vi "AddOrReplaceCmdInCmdList.vi"(7 "CMD LUT in":variant, 8 "error in (no error)":errorcluster, 10 "New Command(s)":string, 11 "Command List In":string) -> (0 "error out":errorcluster, 3 "Command List Out":string, 5 "CMD LUT out":variant)   [LabVIEW 2026, in "MicroPulse_Driver.lvlib"]
uses:
  MicroPulse_Driver.lvlib
  <vilib>/Utility/error.llb/Trim Whitespace One-Sided.vi
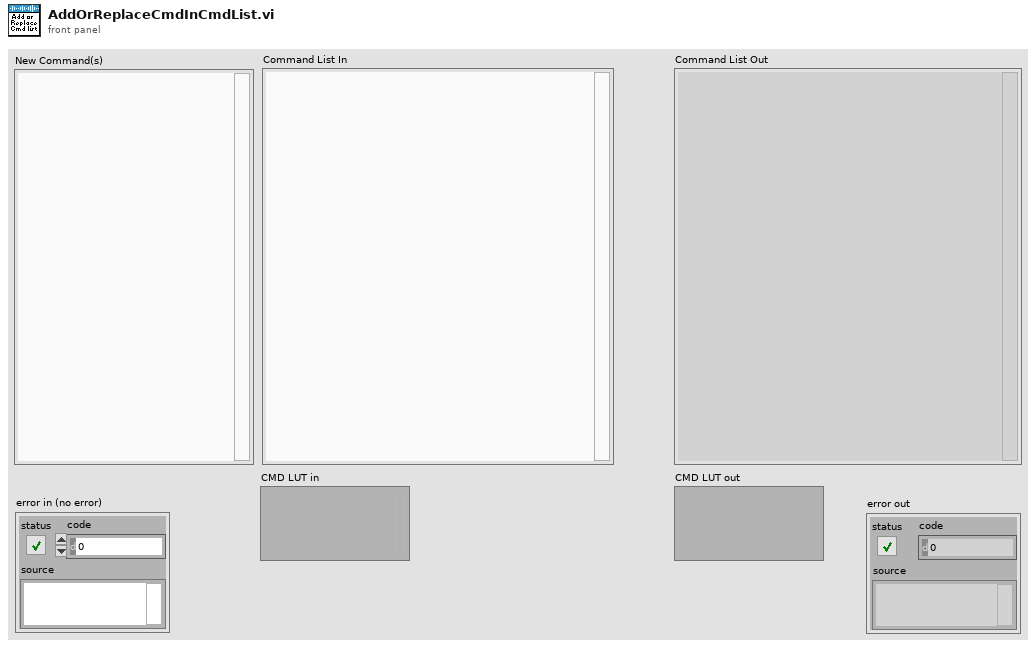
[diagram p1: front panel]
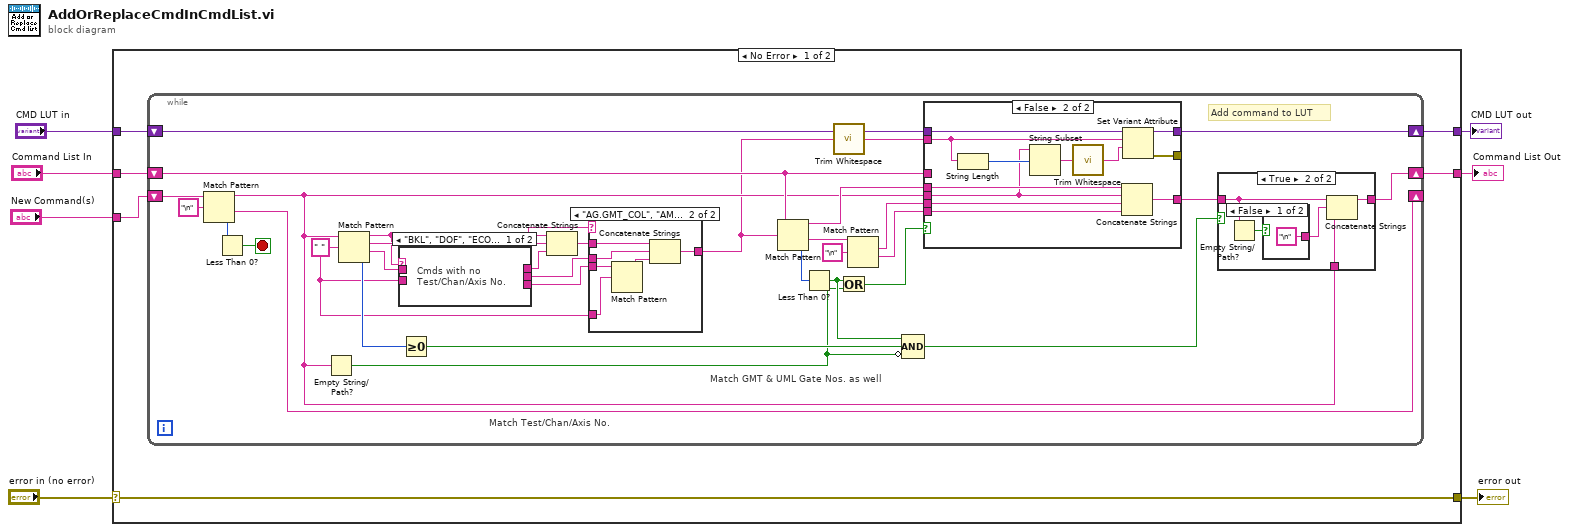
[diagram p0: block diagram]
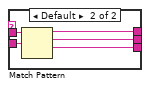
[diagram p2: hidden frame]
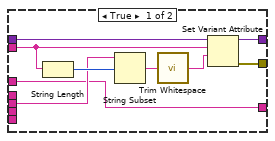
[diagram p6: hidden frame]
diagram:
  n1 = case shown="No Error" "error in (no error)" {
    selector: "error in (no error)" -> [w10 w89]
    tunnel: "Command List In" -> [w13 w88]
    tunnel: [w12 w88] -> w6
    tunnel: "New Command(s)" -> [w11 _]
    tunnel: [w10 w89] -> w3
    tunnel: "CMD LUT in" -> [w9 w87]
    tunnel: [w8 w87] -> w1
    frame No Error {
      n2 = while {
        shift-right: [w38] -> w12
        shift-left: w13 -> [w28]
        shift-right: [w27] -> _
        shift-left: w11 -> [w29]
        shift-right: [w17] -> w8
        shift-left: w9 -> [w18]
        stop <- w30 stop-if-true
        w20 = " " ("regular expression")
        # "Add command to LUT"
        # "Match GMT & UML Gate Nos. as well"
        # "Match Test/Chan/Axis No."
        n3 = Match Pattern(string=w29, regular expression="\n") -> (before substring=w22:string, after substring=w27:string, offset past match=w31:i32)  [unwired: 1 in, 1 out]
        n4 = Less Than 0?(x=w31) -> (x < 0?=w30:bool)
        n5 = Empty String/Path?(string/path=w22) -> (empty?=w34:bool)
        n6 = Match Pattern(string=w22, regular expression=w20) -> (before substring=w15:string, match substring=w24:string, after substring=w26:string, offset past match=w40:i32)  [unwired: 1 in]
        n7 = case shown="\"BKL\", \"DOF\", \"ECON\", \"EMUL\", \"ENCF\", \"ENCM\", \"ENCO\", \"ENCT\", \"FLM\", \"JIT\", \"MPE\", \"NUM\", \"PIG\", \"PRF\", \"SPA\", \"SPQ\", \"SPR\", \"STS\"" w15 {
          tunnel: w26 -> [_ w51]
          tunnel: [_ w50] -> w25
          tunnel: [_ w49] -> w21
          tunnel: w20 -> [_ w48]
          tunnel: [_ w47] -> w19
          frame "BKL", "DOF", "ECON", "EMUL", "ENCF", "ENCM", "ENCO", "ENCT", "FLM", "JIT", "MPE", "NUM", "PIG", "PRF", "SPA", "SPQ", "SPR", "STS" {
            # "Cmds with no\nTest/Chan/Axis No."
          }
          frame Default {
            n8 = Match Pattern(string=w51, regular expression=w48) -> (before substring=w50:string, match substring=w47:string, after substring=w49:string)  [unwired: 1 in, 1 out]
          }
        }
        n9 = Greater Or Equal To 0?(x=w40) -> (x >= 0?=w35:bool)
        n10 = Concatenate Strings(w15, w24, w25) -> (w23:string)
        n11 = case shown="\"AG.GMT_COL\", \"AMM\", \"CML\", \"GIN\", \"GMH\", \"GML\", \"GMT\", \"GTR\", \"HMS\", \"LML\", \"PMG\", \"UML\"" w15 {
          tunnel: [w52 w53] -> w16
          tunnel: w23 -> [w52 w56]
          tunnel: w21 -> [_ w58]
          tunnel: w20 -> [_ w57]
          tunnel: w19 -> [_ w55]
          frame Default {
          }
          frame "AG.GMT_COL", "AMM", "CML", "GIN", "GMH", "GML", "GMT", "GTR", "HMS", "LML", "PMG", "UML" {
            n12 = Match Pattern(string=w58, regular expression=w57) -> (before substring=w54:string)  [unwired: 1 in, 3 out]
            n13 = Concatenate Strings(w56, w55, w54) -> (w53:string)
          }
        }
        n14 = Match Pattern(string=w28, regular expression=w16) -> (before substring=w42:string, after substring=w46:string, offset past match=w41:i32)  [unwired: 1 in, 1 out]
        n15 = Less Than 0?(x=w41) -> (x < 0?=w36:bool)
        n16 = call <vilib>:"Trim Whitespace.vi"("string"=w16) -> ("trimmed string"=w14:string)  [unwired: 1 in]
        n17 = Or(x=w36, y=w34) -> (x .or. y?=w37:bool)
        n18 = Match Pattern(string=w46, regular expression="\n") -> (match substring=w44:string, after substring=w43:string)  [unwired: 1 in, 2 out]
        n19 = Compound Arithmetic op=AND(w36, w35, invert w34) -> (w33:bool)
        n20 = case shown="False" w37 {
          tunnel: w44 -> [_ w82]
          tunnel: w43 -> [_ w86]
          tunnel: w22 -> [w70 w77]
          tunnel: [w68 w85] -> w39
          tunnel: w42 -> [_ w78]
          tunnel: w28 -> [w68 _]
          tunnel: w18 -> [w72 w84]
          tunnel: [w71 w83] -> w17
          tunnel: w14 -> [w69 w80]
          tunnel: [w67 w76] -> _
          frame True {
            n21 = String Length(string=w69) -> (length=w73:i32)
            n22 = String Subset(string=w70, offset (0)=w73) -> (substring=w74:string)  [unwired: 1 in]
            n23 = call <vilib>:"Trim Whitespace.vi"("string"=w74) -> ("trimmed string"=w66:string)  [unwired: 1 in]
            n24 = Set Variant Attribute(Variant=w72, name=w69, value=w66) -> (Variant out=w71:variant, error out=w67:errorcluster)  [unwired: 1 in, 1 out]
          }
          frame False {
            n25 = String Length(string=w80) -> (length=w79:i32)
            n26 = String Subset(string=w77, offset (0)=w79) -> (substring=w81:string)  [unwired: 1 in]
            n27 = call <vilib>:"Trim Whitespace.vi"("string"=w81) -> ("trimmed string"=w75:string)  [unwired: 1 in]
            n28 = Concatenate Strings(w78, w77, w82, w86) -> (w85:string)
            n29 = Set Variant Attribute(Variant=w84, name=w80, value=w75) -> (Variant out=w83:variant, error out=w76:errorcluster)  [unwired: 1 in, 1 out]
          }
        }
        n30 = case shown="True" w33 {
          tunnel: w39 -> [w59 w61]
          tunnel: [w59 w64] -> w38
          tunnel: w22 -> [_ w63]
          frame False {
          }
          frame True {
            n31 = Empty String/Path?(string/path=w61) -> (empty?=w60:bool)
            n32 = case shown="False" w60 {
              tunnel: ["\n" ("string") _] -> w62
              frame False {
              }
              frame True {
              }
            }
            n33 = Concatenate Strings(w61, w62, w63) -> (w64:string)
          }
        }
      }
    }
    frame Error {
    }
  }
  "Command List Out" <- w6
  "error out" <- w3
  "CMD LUT out" <- w1
